vi "Get Localized Phrase Compact Interface 2D.vi"(1 "Key":string[][](array[string])) -> (0 "Translated Phrase":string[][](array[string]))   [LabVIEW 2020]
doc: "Gets the localized phrase by key from the current dictionary.\n\nKey: Unique identifier defined in the dictionary\nTarget Language (current lang): Optional input. Set this to translate a phase to a language other than the current language."
uses:
  Localization FGV Action -- Enum.ctl
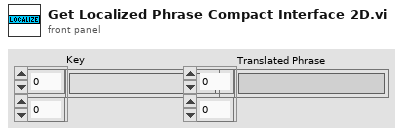
[diagram p1: front panel]
types:
  T1 = typedef "Localization FGV Action -- Enum.ctl" = enum16{"Read Dictionary", "Translate VIs", "Register VI", "Get Languages", "Translate Phrase", "Get Key For Phrase", "Get Phrase For Phrase", "Translate VI", "Unregister"}
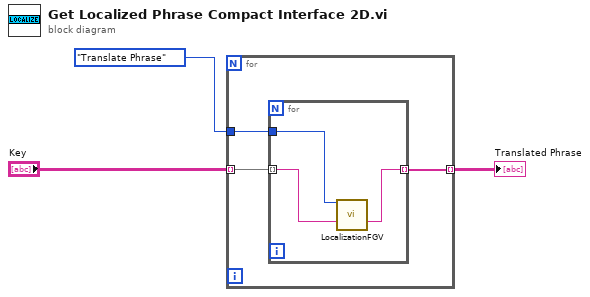
[diagram p0: block diagram]
diagram:
  n1 = for {
    tunnel: Localization_FGV_Action_--_Enum."Translate Phrase" ("Action") -> [w6]
    tunnel: "Key" -> [w5] mode=indexing
    tunnel: [w4] -> w1 mode=indexing
    n2 = for {
      tunnel: w6 -> [w9]
      tunnel: w5 -> [w8] mode=indexing
      tunnel: [w7] -> w4 mode=indexing
      n3 = call "LocalizationFGV.vi"("Action"=w9, "Input"=w8) -> ("Result"=w7:string)  [unwired: 8 in, 5 out]
    }
  }
  "Translated Phrase" <- w1
